vi "ReadReport.vi"(8 "error in (no error)":errorcluster, 11 "FILE PATH TO REPORT DATA":path) -> (0 "error out":errorcluster, 3 "DVR Out":refnum<data-value>)   [LabVIEW 2018, in "Data Operations.lvlib"]
uses:
  Data Operations.lvlib
  Private Controls/Report Data Cluster.ctl
  Private Controls/Data Raw.ctl
  Private Controls/ReadReport States Enum.ctl
  <vilib>/Utility/file.llb/Read Delimited Spreadsheet (string).vi
  <vilib>/Utility/error.llb/Trim Whitespace.vi
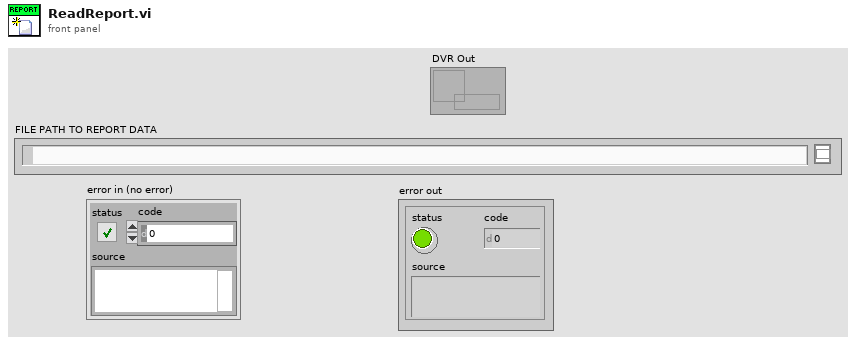
[diagram p1: front panel]
types:
  T1 = typedef "Data Operations.lvlib/ReadReport States Enum.ctl" = enum16{"Initialize", "Read Headers", "Read Raw Data", "Error", "Generate DVR"}
  T2 = typedef "Data Operations.lvlib/Report Data Cluster.ctl" = cluster{"Headers":cluster{"Start Date":timestamp, "End Date":timestamp, "SR Status String":string[], "AE Owner String":string[]}, "Data":T3[]}
  T3 = typedef "Data Operations.lvlib/Data Raw.ctl" = cluster{"SR Number":string, "Status":string, "Summary":string, "AE Owner":string, "AE Group":string, "Contact":string, "SurveyData":cluster{"Resolution Time":dbl, "Total Satisfaction":dbl, "Response Time":dbl, "Courtesy":dbl, "Problem Solved":dbl, "Level of effort":dbl}, "Time Data":cluster{"Last Update Date":timestamp, "Creation Date":timestamp, "Creation week":i16, "Last Update Week":i16, "Creation Year":i16}}
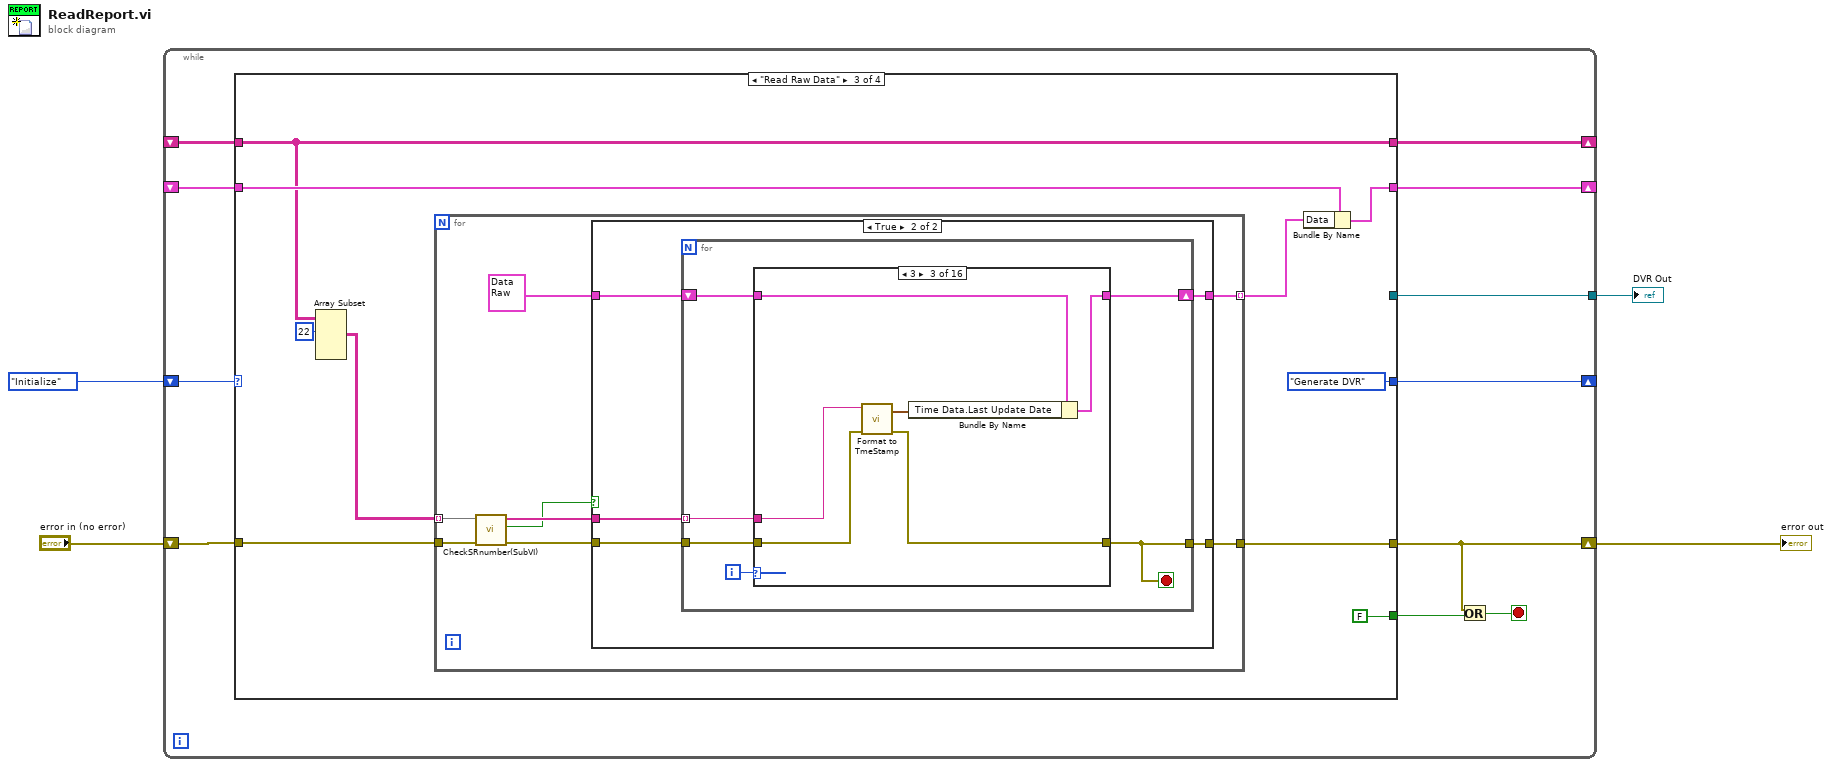
[diagram p0: block diagram]
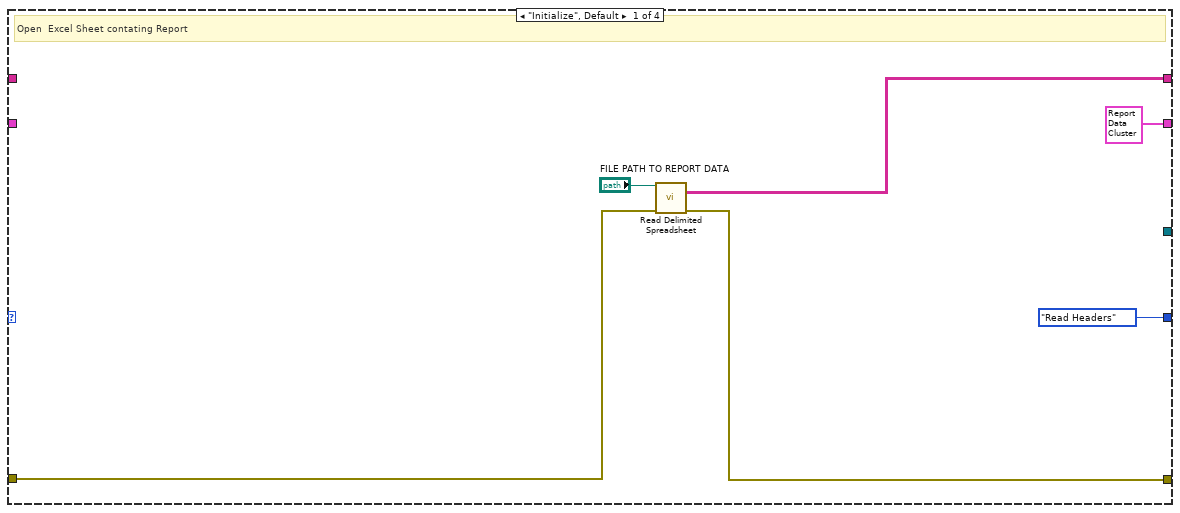
[diagram p2: hidden frame]
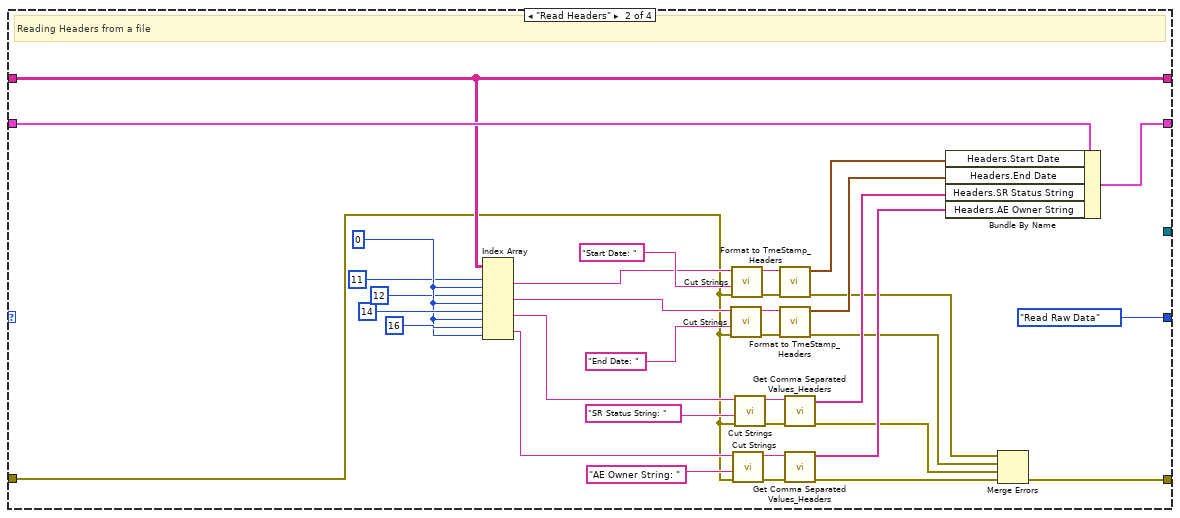
[diagram p3: hidden frame]
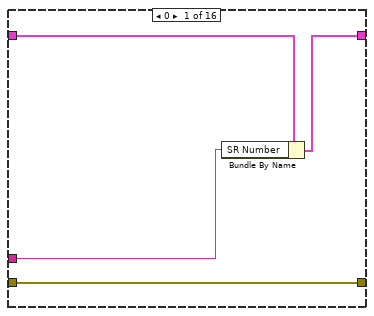
[diagram p5: hidden frame]
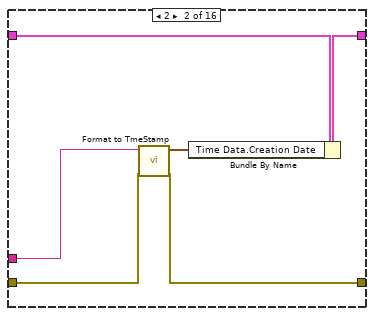
[diagram p6: hidden frame]
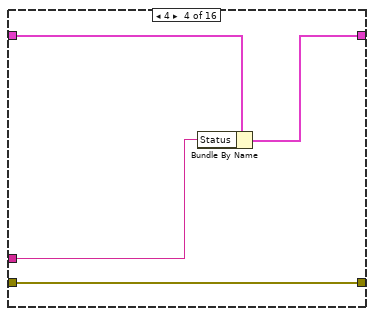
[diagram p7: hidden frame]
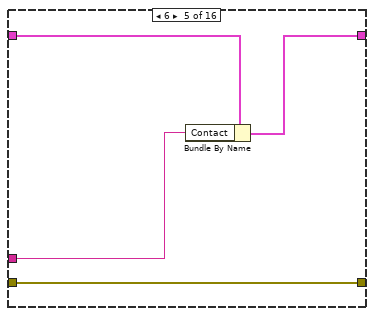
[diagram p8: hidden frame]
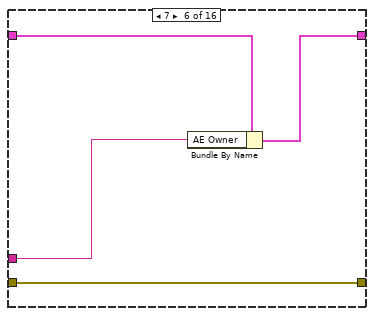
[diagram p9: hidden frame]
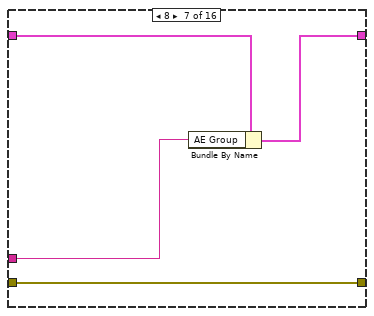
[diagram p10: hidden frame]
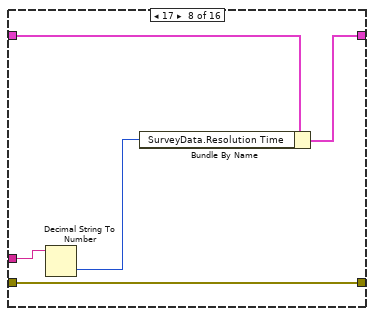
[diagram p11: hidden frame]
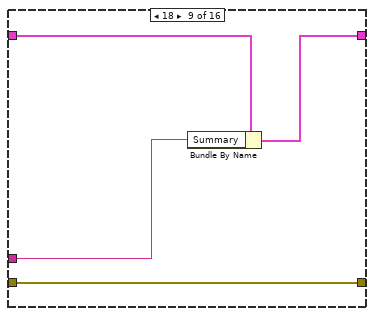
[diagram p12: hidden frame]
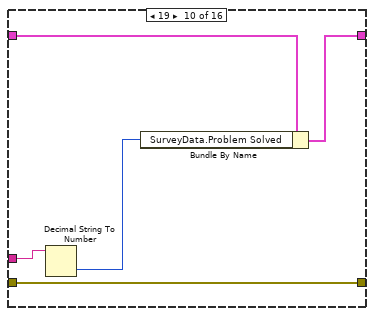
[diagram p13: hidden frame]
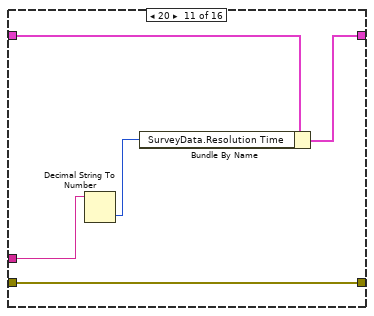
[diagram p14: hidden frame]
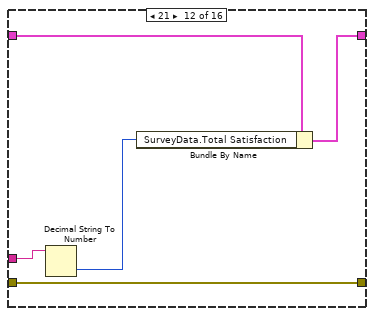
[diagram p15: hidden frame]
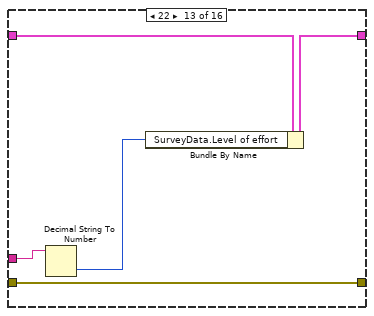
[diagram p16: hidden frame]
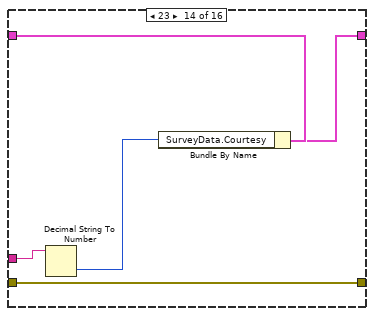
[diagram p17: hidden frame]
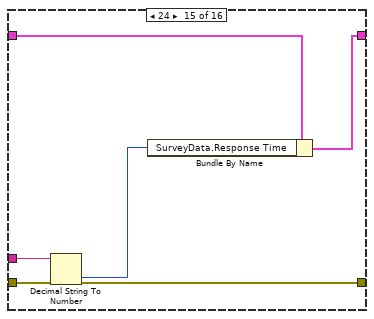
[diagram p18: hidden frame]
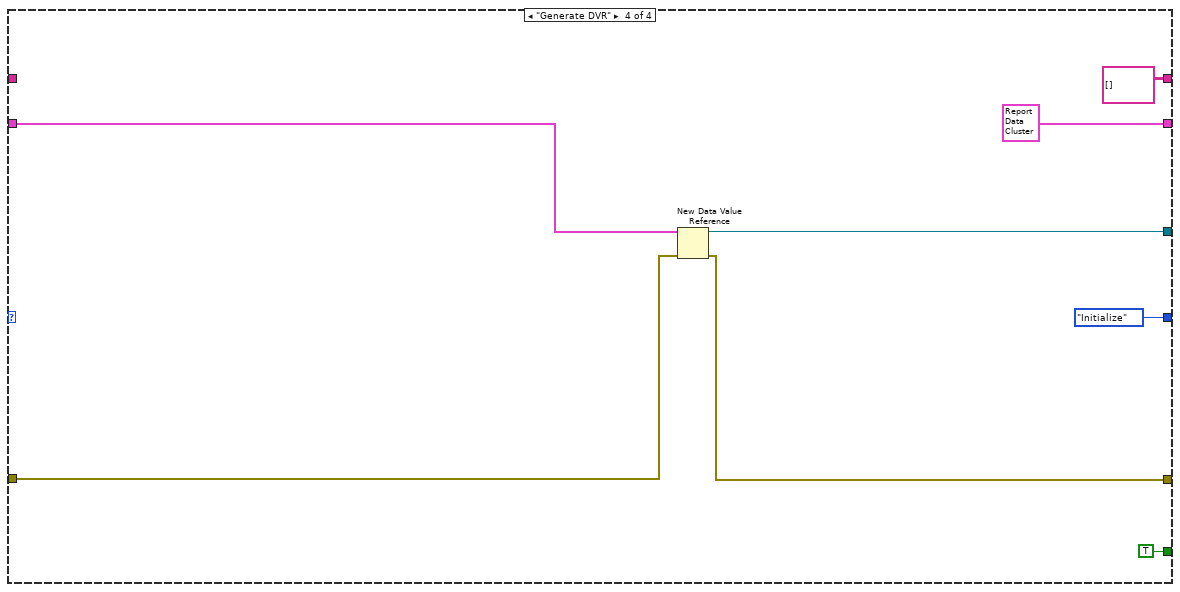
[diagram p20: hidden frame]
diagram:
  n1 = while {
    shift-right: [w6] -> w2
    shift-left: "error in (no error)" -> [w14]
    shift-right: [w12] -> _
    shift-left: _ -> [w13]
    shift-right: [w10] -> _
    shift-left: _ -> [w15]
    shift-right: [w5] -> _
    shift-left: ReadReport_States_Enum."Initialize" -> [w11]
    tunnel: [w9] -> w1
    stop <- w7 stop-if-true
    n2 = case shown="\"Read Raw Data\"" w11 {
      tunnel: w15 -> [_ w29 w57 _]
      tunnel: w14 -> [w17 w28 w61 w167]
      tunnel: [w16 w25 w60 w166] -> w6
      tunnel: w13 -> [_ w32 w66 w168]
      tunnel: [T2 {"Headers"={"Start Date"=timestamp(0 s since 1904-01-01), "End Date"=timestamp(0 s since 1904-01-01), "SR Status String"=[], "AE Owner String"=[]}, "Data"=[]} ("Cluster") w31 w64 T2 {"Headers"={"Start Date"=timestamp(0 s since 1904-01-01), "End Date"=timestamp(0 s since 1904-01-01), "SR Status String"=[], "AE Owner String"=[]}, "Data"=[]} ("Cluster")] -> w12
      tunnel: [w20 w29 w57 string[][] [] ("all rows")] -> w10
      tunnel: [ReadReport_States_Enum."Read Headers" ReadReport_States_Enum."Read Raw Data" ReadReport_States_Enum."Generate DVR" ReadReport_States_Enum."Initialize"] -> w5
      tunnel: [_ _ FALSE TRUE] -> w8
      tunnel: [_ _ _ w165] -> w9
      frame "Initialize", Default {
        # "Open  Excel Sheet contating Report"
        n3 = call-poly <vilib>:"Read Delimited Spreadsheet.vi"("file path (dialog if empty)"="FILE PATH TO REPORT DATA", "error in (no error)"=w17) -> ("all rows"=w20:string[][], "error out"=w16:errorcluster)  [unwired: 8 in, 4 out]
      }
      frame "Read Headers" {
        w46 = 0
        # "Reading Headers from a file"
        n4 = Index Array(array=w29, index (row) #1=11, index (col) #1=w46, index (row) #2=12, index (col) #2=w46, index (row) #3=14 ("disabled index (row)"), index (col) #3=w46, index (row) #4=16 ("disabled index (row)"), index (col) #4=w46) -> (element #1=w37:string, element #2=w45:string, element #3=w50:string, element #4=w55:string)
        n5 = call "Cut Strings.vi"("error in (no error)"=w28, "To Cut"="End Date: ", "Input String"=w45) -> ("error out"=w27:errorcluster, "Output String"=w43:string)  [unwired: 7 in]
        n6 = call "Cut Strings.vi"("error in (no error)"=w28, "To Cut"="Start Date: ", "Input String"=w37) -> ("error out"=w39:errorcluster, "Output String"=w38:string)  [unwired: 7 in]
        n7 = call "Cut Strings.vi"("error in (no error)"=w28, "To Cut"="AE Owner String: ", "Input String"=w55) -> ("error out"=w34:errorcluster, "Output String"=w53:string)  [unwired: 7 in]
        n8 = call "Cut Strings.vi"("error in (no error)"=w28, "To Cut"="SR Status String: ", "Input String"=w50) -> ("error out"=w33:errorcluster, "Output String"=w51:string)  [unwired: 7 in]
        n9 = call "Format to TmeStamp_Headers.vi"("error in"=w39, "String"=w38) -> ("error out"=w22:errorcluster, "Time Stamp Out"=w36:timestamp)  [unwired: 8 in]
        n10 = call "Format to TmeStamp_Headers.vi"("error in"=w27, "String"=w43) -> ("error out"=w23:errorcluster, "Time Stamp Out"=w44:timestamp)  [unwired: 8 in]
        n11 = call "Get Comma Separated Values_Headers.vi"("Error In"=w33, "Output String"=w51) -> ("Error In 2"=w24:errorcluster, "Array"=w52:string[])  [unwired: 8 in]
        n12 = call "Get Comma Separated Values_Headers.vi"("Error In"=w34, "Output String"=w53) -> ("Error In 2"=w26:errorcluster, "Array"=w56:string[])  [unwired: 8 in]
        n13 = Bundle By Name(cluster=w32, "Headers.Start Date"=w36, "Headers.End Date"=w44, "Headers.SR Status String"=w52, "Headers.AE Owner String"=w56) -> (w31:T2)
        n14 = Merge Errors(w22, w23, w24, w26) -> (w25:errorcluster)
      }
      frame "Read Raw Data" {
        n15 = Array Subset(array=w57, index (row)=22 ("index")) -> (w62:string[][])  [unwired: 3 in]
        n16 = for {
          tunnel: w62 -> [w72] mode=indexing
          tunnel: [w74] -> w65 mode=indexing
          tunnel: w61 -> [w71]
          tunnel: [w73] -> w60
          n17 = call "CheckSRnumber(SubVI).vi"("error in (no error)"=w71, "Data In"=w72) -> ("error out"=w70:errorcluster, "Valid ?"=w67:bool, "Data Out"=w69:string[])  [unwired: 7 in]
          n18 = case shown="True" w67 {
            tunnel: [w76 w81] -> w74
            tunnel: [w75 w80] -> w73
            tunnel: w70 -> [w75 w79]
            tunnel: w69 -> [_ w78]
            tunnel: T3 {"SR Number"="", "Status"="", "Summary"="", "AE Owner"="", "AE Group"="", "Contact"="", "SurveyData"={"Resolution Time"=0.0, "Total Satisfaction"=0.0, "Response Time"=0.0, "Courtesy"=0.0, "Problem Solved"=0.0, "Level of effort"=0.0}, "Time Data"={"Last Update Date"=timestamp(0 s since 1904-01-01), "Creation Date"=timestamp(0 s since 1904-01-01), "Creation week"=0, "Last Update Week"=0, "Creation Year"=0}} ("Cluster") -> [w76 w77]
            frame False {
            }
            frame True {
              n19 = for {
                tunnel: w78 -> [w85] mode=indexing
                shift-right: [w86] -> w81
                shift-left: w77 -> [w87]
                tunnel: w79 -> [w83]
                tunnel: [w82] -> w80
                i -> [w84]
                stop <- w82 stop-if-true
                n20 = case shown="3" w84 {
                  tunnel: w87 -> [w91 w97 w103 w107 w110 w115 w119 w124 w128 w133 w138 w143 w148 w153 w155 w160]
                  tunnel: [w90 w96 w102 w106 w108 w114 w118 w123 w127 w132 w137 w142 w147 w152 w154 w160] -> w86
                  tunnel: w85 -> [w89 w94 w100 w105 w109 w113 w117 w121 w125 w130 w135 w140 w145 w150 w157 _]
                  tunnel: w83 -> [w88 w93 w99 w104 w111 w112 w116 w122 w126 w131 w136 w141 w146 w151 w156 w159]
                  tunnel: [w88 w92 w98 w104 w111 w112 w116 w122 w126 w131 w136 w141 w146 w151 w156 w159] -> w82
                  frame 0 {
                    n21 = Bundle By Name(cluster=w91, "SR Number"=w89) -> (w90:T3)
                  }
                  frame 2 {
                    n22 = call "Format to TmeStamp.vi"("error in"=w93, "String"=w94) -> ("error out"=w92:errorcluster, "Time Stamp"=w95:timestamp)  [unwired: 8 in]
                    n23 = Bundle By Name(cluster=w97, "Time Data.Creation Date"=w95) -> (w96:T3)
                  }
                  frame 3 {
                    n24 = call "Format to TmeStamp.vi"("error in"=w99, "String"=w100) -> ("error out"=w98:errorcluster, "Time Stamp"=w101:timestamp)  [unwired: 8 in]
                    n25 = Bundle By Name(cluster=w103, "Time Data.Last Update Date"=w101) -> (w102:T3)
                  }
                  frame 4 {
                    n26 = Bundle By Name(cluster=w107, "Status"=w105) -> (w106:T3)
                  }
                  frame 6 {
                    n27 = Bundle By Name(cluster=w110, "Contact"=w109) -> (w108:T3)
                  }
                  frame 7 {
                    n28 = Bundle By Name(cluster=w115, "AE Owner"=w113) -> (w114:T3)
                  }
                  frame 8 {
                    n29 = Bundle By Name(cluster=w119, "AE Group"=w117) -> (w118:T3)
                  }
                  frame 17 {
                    n30 = Decimal String To Number(string=w121) -> (number=w120:i32)  [unwired: 2 in, 1 out]
                    n31 = Bundle By Name(cluster=w124, "SurveyData.Resolution Time"=w120) -> (w123:T3)
                  }
                  frame 18 {
                    n32 = Bundle By Name(cluster=w128, "Summary"=w125) -> (w127:T3)
                  }
                  frame 19 {
                    n33 = Decimal String To Number(string=w130) -> (number=w129:i32)  [unwired: 2 in, 1 out]
                    n34 = Bundle By Name(cluster=w133, "SurveyData.Problem Solved"=w129) -> (w132:T3)
                  }
                  frame 20 {
                    n35 = Decimal String To Number(string=w135) -> (number=w134:i32)  [unwired: 2 in, 1 out]
                    n36 = Bundle By Name(cluster=w138, "SurveyData.Resolution Time"=w134) -> (w137:T3)
                  }
                  frame 21 {
                    n37 = Decimal String To Number(string=w140) -> (number=w139:i32)  [unwired: 2 in, 1 out]
                    n38 = Bundle By Name(cluster=w143, "SurveyData.Total Satisfaction"=w139) -> (w142:T3)
                  }
                  frame 22 {
                    n39 = Decimal String To Number(string=w145) -> (number=w144:i32)  [unwired: 2 in, 1 out]
                    n40 = Bundle By Name(cluster=w148, "SurveyData.Level of effort"=w144) -> (w147:T3)
                  }
                  frame 23 {
                    n41 = Decimal String To Number(string=w150) -> (number=w149:i32)  [unwired: 2 in, 1 out]
                    n42 = Bundle By Name(cluster=w153, "SurveyData.Courtesy"=w149) -> (w152:T3)
                  }
                  frame 24 {
                    n43 = Decimal String To Number(string=w157) -> (number=w158:i32)  [unwired: 2 in, 1 out]
                    n44 = Bundle By Name(cluster=w155, "SurveyData.Response Time"=w158) -> (w154:T3)
                  }
                  frame Default {
                  }
                }
              }
            }
          }
        }
        n45 = Bundle By Name(cluster=w66, "Data"=w65) -> (w64:T2)
      }
      frame "Generate DVR" {
        n46 = New Data Value Reference(data value=w168, error in=w167) -> (data value reference=w165:refnum<data-value>, error out=w166:errorcluster)
      }
    }
    n47 = Or(x=w6, y=w8) -> (x .or. y?=w7:bool)
  }
  "error out" <- w2
  "DVR Out" <- w1
